vi "004JohnsDay.vi"() -> ()   [LabVIEW 2010]
panel:
  out "johnsLightIsOn":bool
  in  "Time of day":dbl(slide) scale=0.0..24.0
  # "[Johns light]"
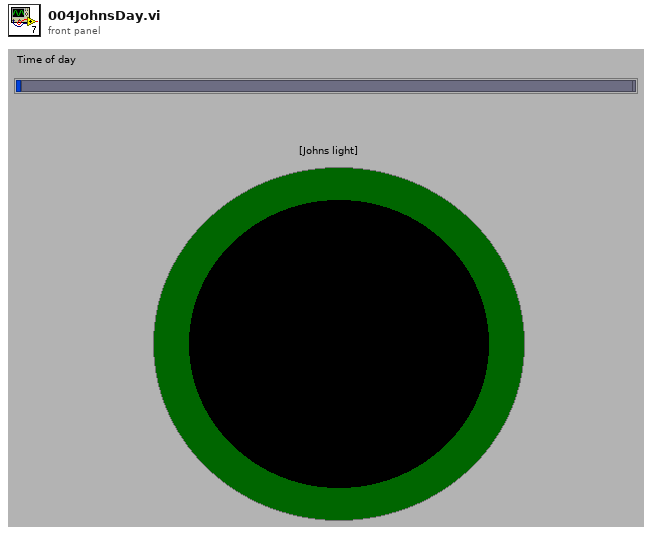
[diagram p1: front panel]
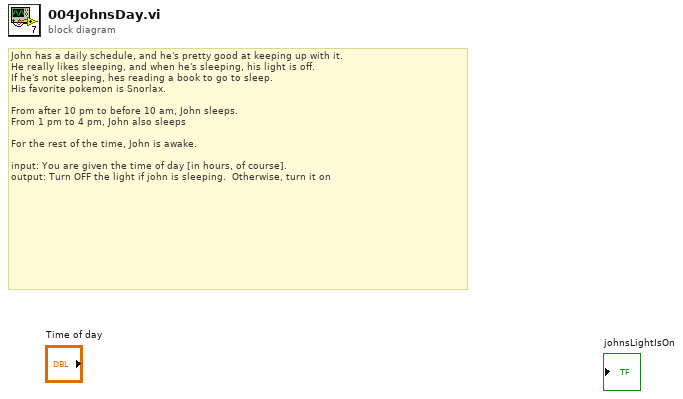
[diagram p0: block diagram]
diagram:
  # "John has a daily schedule, and he's pretty good at keeping up with it.\nHe really likes sleeping, and when he's sleeping, his light is off.  \nIf he's not sleeping, hes reading a book to go to sleep.\nHis favorite pokemon is Snorlax.\n\nFrom after 10 pm to before 10 am, John sleeps.\nFrom 1 pm to 4 pm, John also sleeps\n\nFor the rest of the time, John is awake.\n\ninput: You are given the time of day [in hours, of course].  \noutput: Turn OFF the light if john is sleeping.  Otherwise, turn it on"
